vi "SC_States_For_Seek_Sub_VI.vi"() -> (2 "Array":dbl[](array[numeric]), 3 "SC States for Weld":dbl[](array[numeric]))   [LabVIEW 2017]
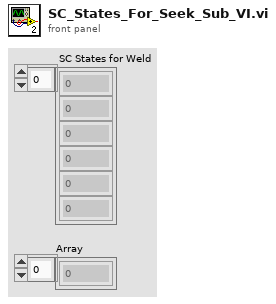
[diagram p1: front panel]
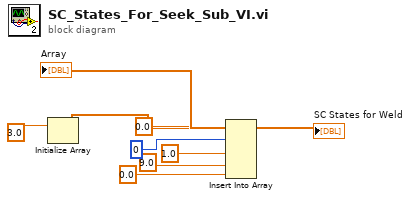
[diagram p0: block diagram]
diagram:
  n1 = Initialize Array(3.0 ("element")) -> (w2:dbl[])  [unwired: 1 in]
  n2 = Insert Into Array(array=w2, index=0, new element #1=0.0 ("new element/subarray"), new element #2=1.0 ("new element/subarray"), new element #3=9.0 ("new element/subarray"), new element #4=0.0 ("new element/subarray")) -> (→"SC States for Weld" →"Array":dbl[])
